vi "Parse IDN.vi"(8 "error in (no error)":errorcluster, 11 "*IDN?":string) -> (0 "error out":errorcluster, 1 "Serial Number":string, 2 "Model":string, 4 "Firmware (Major.Minor.Release)":string, 5 "Manufacturer":string)   [LabVIEW 2019, in "RP100.lvlib"]
uses:
  RP100.lvlib
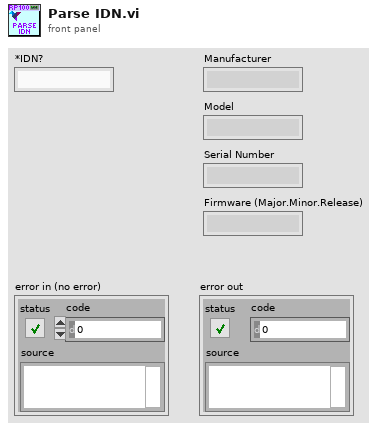
[diagram p1: front panel]
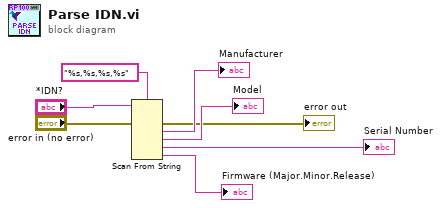
[diagram p0: block diagram]
diagram:
  n1 = Scan From String(format string="%s,%s,%s,%s", input string="*IDN?", error in="error in (no error)") -> (error out=→"error out":errorcluster, output 1=→"Manufacturer":string, output 2=→"Model":string, output 3=→"Serial Number":string, output 4=→"Firmware (Major.Minor.Release)":string)  [unwired: 5 in, 2 out]
